vi "Match Cfg to Hardware.vi"(7 "FP Ctrls":refnum<class "FP Controls.lvclass">, 8 "error in":errorcluster, 10 "selected path":path, 11 "Cfg wChassis":T1) -> (0 "error out":errorcluster, 1 "HW Error?":bool, 3 "Cfg wChassis":T1)   [LabVIEW 2018, in "Configuration Grandmaster.lvlib" / "Cfg Grandmaster.lvclass"]
uses:
  Cfg Grandmaster.lvclass
  Custom Ctrls/Master Cfg/ge_Cfg wChassis.ctl
  Class Chassis Cfg/ChassisCfg.lvclass
  Class Chassis BOM/Chassis BOM.lvclass
  Data Acquisition/Class Chassis Tasks/Chassis Tasks.lvclass
  Class FP Ctrls/FP Controls.lvclass
  Class Chassis BOM/Chassis BOM.lvclass/Chassis BOM.ctl
  Common/Controls/TE_Designator.ctl
  Class Chassis BOM/Read ChassisType.vi
  Class Chassis BOM/Write CfgFile.vi
  Class Chassis BOM/Write HW Mods.vi
  Class Timing Group/TimingGrp.lvclass
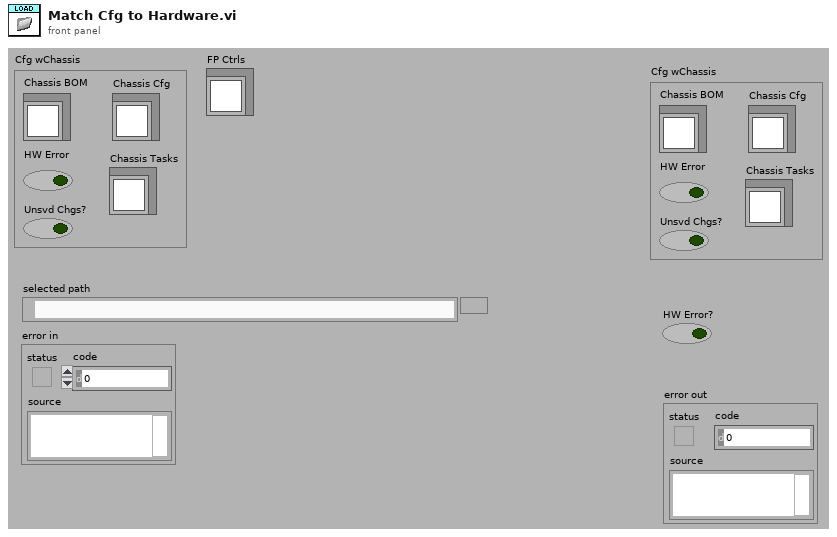
[diagram p1: front panel]
types:
  T1 = typedef "ge_Cfg wChassis.ctl" = cluster{"Chassis BOM":refnum<class "Chassis BOM.lvclass">, "Chassis Cfg":refnum<class "ChassisCfg.lvclass">, "Chassis Tasks":refnum<class "Chassis Tasks.lvclass">, "HW Error":bool, "Unsvd Chgs?":bool}
  T2 = typedef "Chassis Type.ctl" = enum16{"Not Supported", "C Series 1-Slot", "C Series 4-Slot", "C Series 8-Slot", "PXI 8-Slot", "PXIe 18-Slot"}
  T3 = typedef "TE_Designator.ctl" = enum16{"High Speed", "Low Speed"}
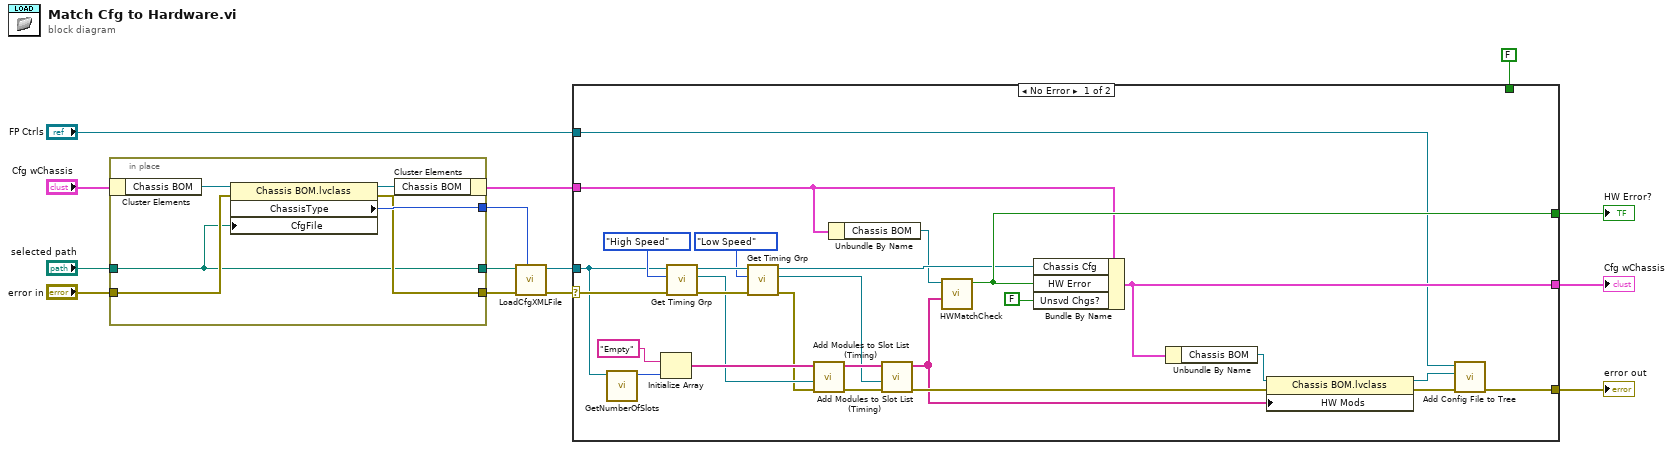
[diagram p0: block diagram]
diagram:
  n1 = in-place {
    in-place-border: [w20] -> w9
    in-place-border: [w19] -> w8
    in-place-border: "error in" -> [w18]
    in-place-border: "selected path" -> [w15]
    in-place-border: [w15] -> w3
    n2 = in-place-cluster #1("Cfg wChassis") -> ("Chassis BOM"=w17:refnum<class "Chassis BOM.lvclass">)
    n3 = property class="Chassis BOM.lvclass"(reference=w17, error in=w18, "CfgFile"=w15) -> (reference out=w16:refnum<class "Chassis BOM.lvclass">, error out=w19:errorcluster, "ChassisType"=w20:T2)
    n4 = in-place-cluster #1("Chassis BOM"=w16) -> (w4:T1)
  }
  n5 = call "LoadCfgXMLFile.vi"("ChassisType"=w9, "error in"=w8, "XML File Path"=w3) -> ("error out"=w11:errorcluster, "Chassis Cfg"=w10:refnum<class "ChassisCfg.lvclass">)  [unwired: 7 in]
  n6 = case shown="No Error" w11 {
    selector: w11 -> [w36 w50]
    tunnel: [w28 w49] -> w14
    tunnel: [w25 w50] -> w13
    tunnel: w4 -> [w22 w49]
    tunnel: [w47 w48] -> w12
    tunnel: w10 -> [w31 _]
    tunnel: "FP Ctrls" -> [w23 _]
    tunnel: FALSE ("HW Error?") -> [_ w48]
    frame No Error {
      n7 = call "GetNumberOfSlots.vi"("Chassis Cfg"=w31) -> ("# of Slots"=w43:i32)  [unwired: 10 in]
      n8 = Initialize Array("Empty", w43) -> (w44:string[])
      n9 = call "Get Timing Grp.vi"("error in (no error)"=w36, "Timing Engine"=TE_Designator."High Speed", "Chassis Cfg"=w31) -> ("error out"=w39:errorcluster, "Timing Groups"=w38:refnum<class "TimingGrp.lvclass">, "Chassis Cfg"=w35:refnum<class "ChassisCfg.lvclass">)  [unwired: 6 in]
      n10 = call "Get Timing Grp.vi"("error in (no error)"=w39, "Timing Engine"=TE_Designator."Low Speed", "Chassis Cfg"=w35) -> ("error out"=w37:errorcluster, "Timing Groups"=w40:refnum<class "TimingGrp.lvclass">, "Chassis Cfg"=w34:refnum<class "ChassisCfg.lvclass">)  [unwired: 6 in]
      n11 = call "Add Modules to Slot List (Timing).vi"("error in (no error)"=w37, "TimingGrp in"=w38, "SlotMod List"=w44) -> ("error out"=w41:errorcluster, "Slot Mod Lilst"=w45:string[])  [unwired: 7 in]
      n12 = Unbundle By Name(w22) -> ("Chassis BOM"=w21:refnum<class "Chassis BOM.lvclass">)
      n13 = call "Add Modules to Slot List (Timing).vi"("error in (no error)"=w41, "TimingGrp in"=w40, "SlotMod List"=w45) -> ("error out"=w30:errorcluster, "Slot Mod Lilst"=w29:string[])  [unwired: 7 in]
      n14 = call "HWMatchCheck.vi"("File Mods"=w29, "Chassis BOM"=w21) -> ("HW Error?"=w47:bool)  [unwired: 9 in]
      n15 = Bundle By Name(cluster=w22, "Chassis Cfg"=w34, "HW Error"=w47, "Unsvd Chgs?"=FALSE) -> (w28:T1)
      n16 = Unbundle By Name(w28) -> ("Chassis BOM"=w27:refnum<class "Chassis BOM.lvclass">)
      n17 = property class="Chassis BOM.lvclass"(reference=w27, error in=w30, "HW Mods"=w29) -> (reference out=w24:refnum<class "Chassis BOM.lvclass">, error out=w26:errorcluster)
      n18 = call "Add Config File to Tree.vi"("error in"=w26, "HW Chassis List"=w24, "FP Controls in"=w23) -> ("error out"=w25:errorcluster)  [unwired: 7 in, 1 out]
    }
    frame Error {
    }
  }
  "Cfg wChassis" <- w14
  "error out" <- w13
  "HW Error?" <- w12
